vi "Server_test.vi"() -> ()   [LabVIEW 2021]
uses:
  <vilib>/numeric/Random Number (Range) DBL.vi
panel:
  out "hex of float":string
  out "length":string
  out "number\ngenerated":dbl
  out "Unusued":string
  out "*(type *) &x":string
  out "Iteration":i32
  out "Command\nreceived":string
  out "error out":errorcluster
  out "String":string
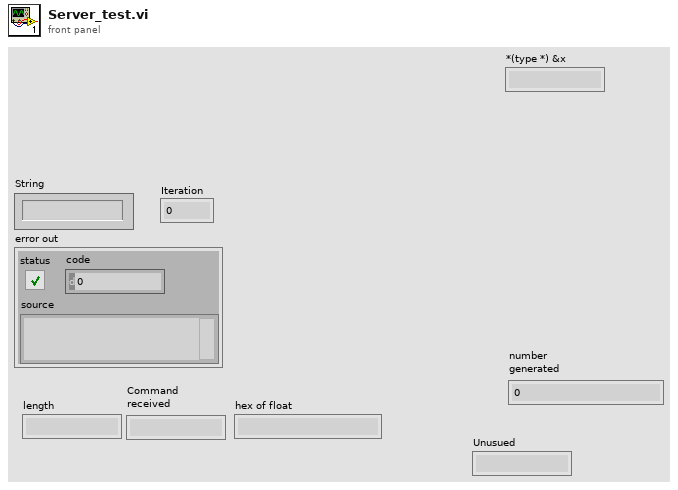
[diagram p1: front panel]
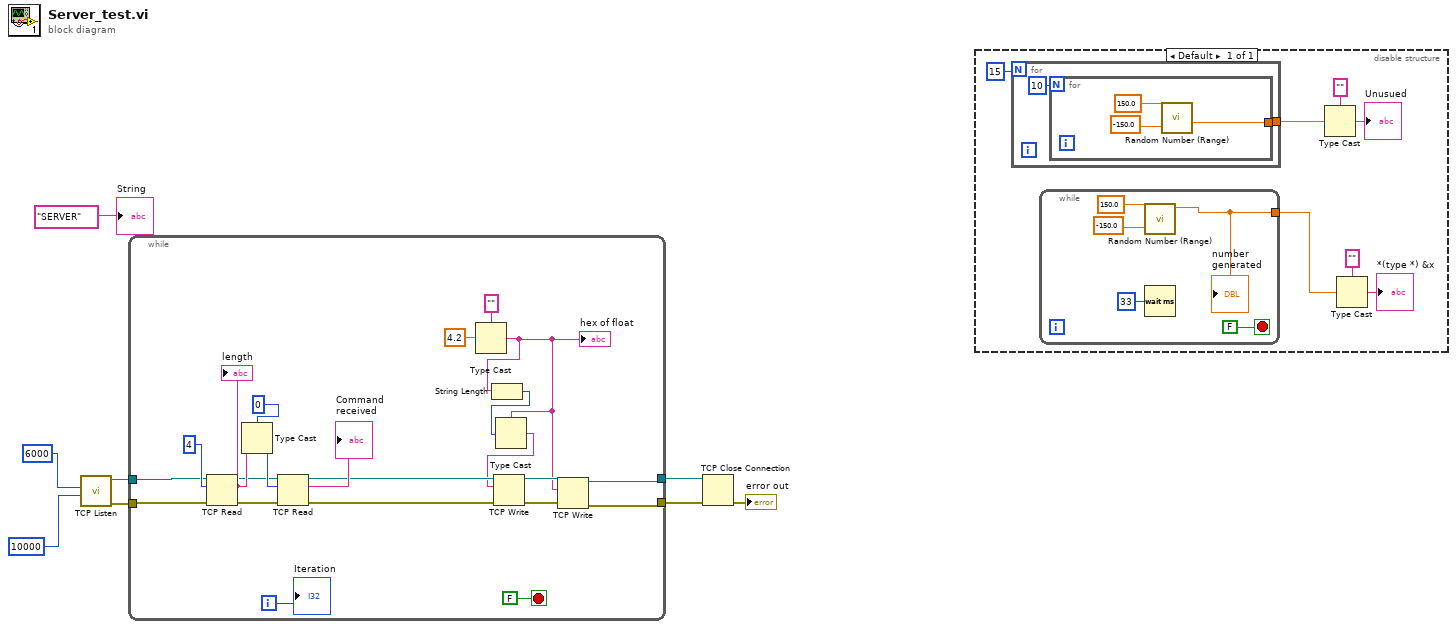
[diagram p0: block diagram]
diagram:
  n1 = call <vilib>:"TCP Listen.vi"("timeout ms (wait forever: -1)"=10000, "port"=u16 6000) -> ("error out"=w2:errorcluster, "connection ID"=w1:refnum<k5>)  [unwired: 5 in, 3 out]
  n2 = while {
    tunnel: [w14] -> w7
    tunnel: [w13] -> w6
    tunnel: w2 -> [w24]
    tunnel: w1 -> [w22]
    i -> [w19]
    stop <- FALSE stop-if-true
    n3 = TCP Read(connection ID=w22, bytes to read=4, error in (no error)=w24) -> (connection ID out=w28:refnum<k5>, data out=w29:string, error out=w26:errorcluster)  [unwired: 2 in]
    "length" <- w29
    n4 = Type Cast(type=0, x=w29) -> (*(type *) &x=w30:i32)
    n5 = TCP Read(connection ID=w28, bytes to read=w30, error in (no error)=w26) -> (connection ID out=w20:refnum<k5>, data out=→"Command\nreceived":string, error out=w21:errorcluster)  [unwired: 2 in]
    n6 = Type Cast(type="", x=4.2) -> (*(type *) &x=w10:string)
    "hex of float" <- w10
    n7 = String Length(string=w10) -> (length=w11:i32)
    n8 = Type Cast(type=w10, x=w11) -> (*(type *) &x=w9:string)
    n9 = TCP Write(connection ID=w20, data in=w9, error in (no error)=w21) -> (connection ID out=w15:refnum<k5>, error out=w12:errorcluster)  [unwired: 1 in, 1 out]
    n10 = TCP Write(connection ID=w15, data in=w10, error in (no error)=w12) -> (connection ID out=w14:refnum<k5>, error out=w13:errorcluster)  [unwired: 1 in, 1 out]
    "Iteration" <- w19
  }
  n11 = TCP Close Connection(connection ID=w7, error in (no error)=w6) -> (error out=→"error out":errorcluster)  [unwired: 1 in, 1 out]
  n12 = disable-structure shown="Default" {
    frame Enabled {
      n13 = for {
        N: 15 -> [_]
        tunnel: [w44] -> w36
        n14 = for {
          N: 10 -> [_]
          tunnel: [w45] -> w44
          n15 = call-poly <vilib>:"Random Number (Range).vi"("lower bound (0)"=-150.0, "upper bound (100)"=150.0) -> ("number"=w45:dbl)  [unwired: 9 in]
        }
      }
      n16 = while {
        tunnel: [w38] -> w32
        stop <- FALSE stop-if-true
        n17 = call-poly <vilib>:"Random Number (Range).vi"("lower bound (0)"=-150.0, "upper bound (100)"=150.0) -> ("number"=w38:dbl)  [unwired: 9 in]
        "number\ngenerated" <- w38
        n18 = Wait (ms)(milliseconds to wait=u32 33) -> ()  [unwired: 1 out]
      }
      n19 = Type Cast(type="", x=w36) -> (*(type *) &x=→"Unusued":string)
      n20 = Type Cast(type="", x=w32) -> (*(type *) &x=→"*(type *) &x":string)
    }
  }
  "String" <- "SERVER" ("String")
